vi "TEST Set Key Value (RAW).vi"() -> ()   [LabVIEW 2013, in "Carya Config.lvclass"]
doc: "Copyright 2018, Carya Automatisering, Wiebe Walstra."
uses:
  Carya Config.lvclass
panel:
  out "String":string="[section 1]\nkey 1=2\nkey 2=2\nkey 3=2\nkey 4=2\n\nkey 7=2\r\nkey 8=2\r\n[section 2]\ngdfgsd=32\r\n[section 3]\r\nkey 12=2"
  out "value written?":bool[](array[boolean])=[TRUE, TRUE, TRUE, TRUE, FALSE, FALSE, TRUE, TRUE, FALSE, FALSE, FALSE, TRUE]
  out "created key?":bool[](array[boolean])=[FALSE, FALSE, FALSE, FALSE, FALSE, FALSE, TRUE, TRUE, FALSE, FALSE, FALSE, TRUE]
  out "created session?":bool[](array[boolean])=[FALSE, FALSE, FALSE, FALSE, FALSE, FALSE, FALSE, FALSE, FALSE, FALSE, FALSE, TRUE]
  # "Should return the values that are set as defaults."
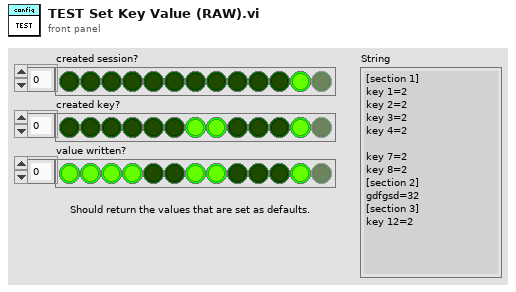
[diagram p1: front panel]
types:
  T1 = cluster{"Section":string, "Key":string, "session?":bool, "key?":bool, "value":string}[]
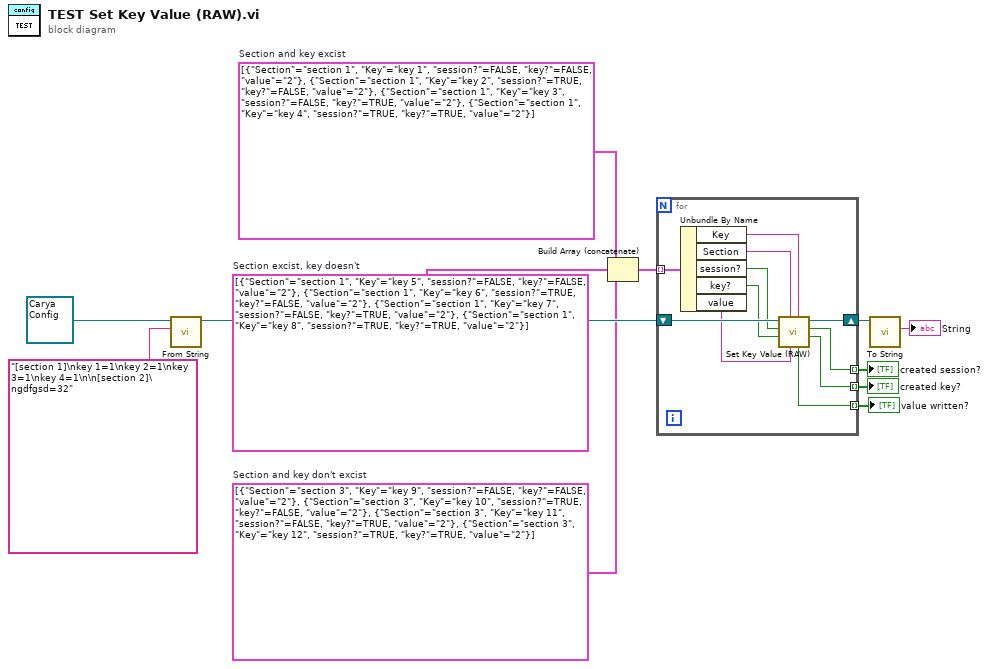
[diagram p0: block diagram]
diagram:
  w4 = T1 [{"Section"="section 3", "Key"="key 9", "session?"=FALSE, "key?"=FALSE, "value"="2"}, {"Section"="section 3", "Key"="key 10", "session?"=TRUE, "key?"=FALSE, "value"="2"}, {"Section"="section 3", "Key"="key 11", "session?"=FALSE, "key?"=TRUE, "value"="2"}, {"Section"="section 3", "Key"="key 12", "session?"=TRUE, "key?"=TRUE, "value"="2"}]  # Section and key don't excist
  w1 = T1 [{"Section"="section 1", "Key"="key 5", "session?"=FALSE, "key?"=FALSE, "value"="2"}, {"Section"="section 1", "Key"="key 6", "session?"=TRUE, "key?"=FALSE, "value"="2"}, {"Section"="section 1", "Key"="key 7", "session?"=FALSE, "key?"=TRUE, "value"="2"}, {"Section"="section 1", "Key"="key 8", "session?"=TRUE, "key?"=TRUE, "value"="2"}]  # Section excist, key doesn't
  w2 = T1 [{"Section"="section 1", "Key"="key 1", "session?"=FALSE, "key?"=FALSE, "value"="2"}, {"Section"="section 1", "Key"="key 2", "session?"=TRUE, "key?"=FALSE, "value"="2"}, {"Section"="section 1", "Key"="key 3", "session?"=FALSE, "key?"=TRUE, "value"="2"}, {"Section"="section 1", "Key"="key 4", "session?"=TRUE, "key?"=TRUE, "value"="2"}]  # Section and key excist
  n1 = call-dynamic "From String.vi"("String"="[section 1]\nkey 1=1\nkey 2=1\nkey 3=1\nkey 4=1\n\n[section 2]\ngdfgsd=32", "Carya Config in"=refnum<class "Carya Config.lvclass"> refnum) -> ("Carya Config out"=w10:refnum<class "Carya Config.lvclass">)  [unwired: 7 in, 2 out]
  n2 = Build Array (concatenate)(w2, w1, w4) -> (w3:T1)
  n3 = for {
    shift-right: [w22] -> w6
    shift-left: w10 -> [w23]
    tunnel: [w21] -> w9 mode=indexing
    tunnel: [w20] -> w8 mode=indexing
    tunnel: [w19] -> w7 mode=indexing
    tunnel: w3 -> [w13] mode=indexing
    n4 = Unbundle By Name(w13) -> ("Key"=w17:string, "Section"=w18:string, "session?"=w16:bool, "key?"=w15:bool, "value"=w14:string)
    n5 = call-dynamic "Set Key Value (RAW).vi"("Key name"=w17, "Key value"=w14, "Section name"=w18, "Create key? [T]"=w15, "Create section? [T]"=w16, "Carya Config in"=w23) -> ("Created key?"=w20:bool, "Created session?"=w21:bool, "Carya Config out"=w22:refnum<class "Carya Config.lvclass">, "Value written?"=w19:bool)  [unwired: 1 in, 1 out]
  }
  "created session?" <- w9
  "created key?" <- w8
  "value written?" <- w7
  n6 = call-dynamic "To String.vi"("Carya Config in"=w6) -> ("String"=→"String":string)  [unwired: 8 in, 2 out]
